vi "ExFilterWheelIN.vi"() -> ()   [LabVIEW 2010]
panel:
  out "Number of Filter Wheels":i16
  in  "?":bool
  out "Filter Wheel Open":bool
  out "Number Of Filters":i16=1 min=1 step=1
  in  "?":bool
  in  "?":bool
  out "Filter":i16=1 min=0 step=1
  in  "?":bool
  in  "?":bool
  in  "?":bool
  in  "Filter":i16=1 min=1 max=100 step=1
  out "error out":errorcluster
  in  "error in":errorcluster
  # "ExFilterWheelIN.vi (InSpectrum Only)\nThis example shows how access a filter wheel on the InSpectrum.\nNot all commands may be available for all filter wheels.\nNOTE: The properly configured spectrometer .ini file must be\npresent in the LabVIEW folder for spectrometer operation."
  # "Currently, there is only 1 filter wheel\navailable on the InSpectrum."
  # "The number of filters is set in the .ini file"
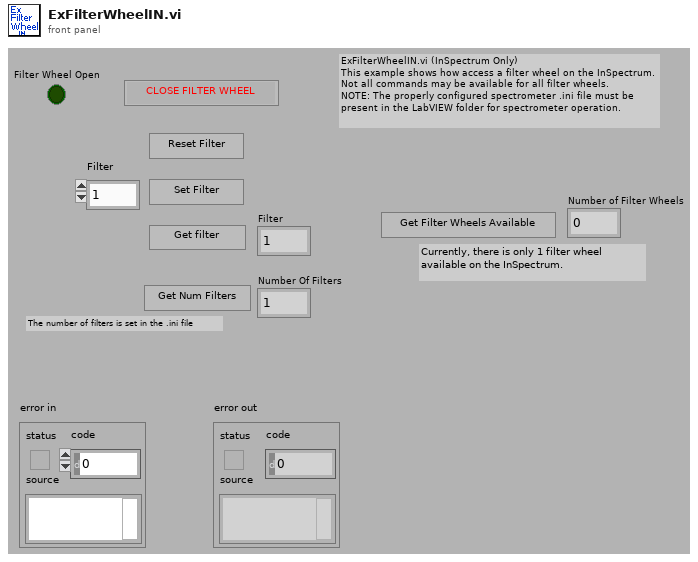
[diagram p1: front panel]
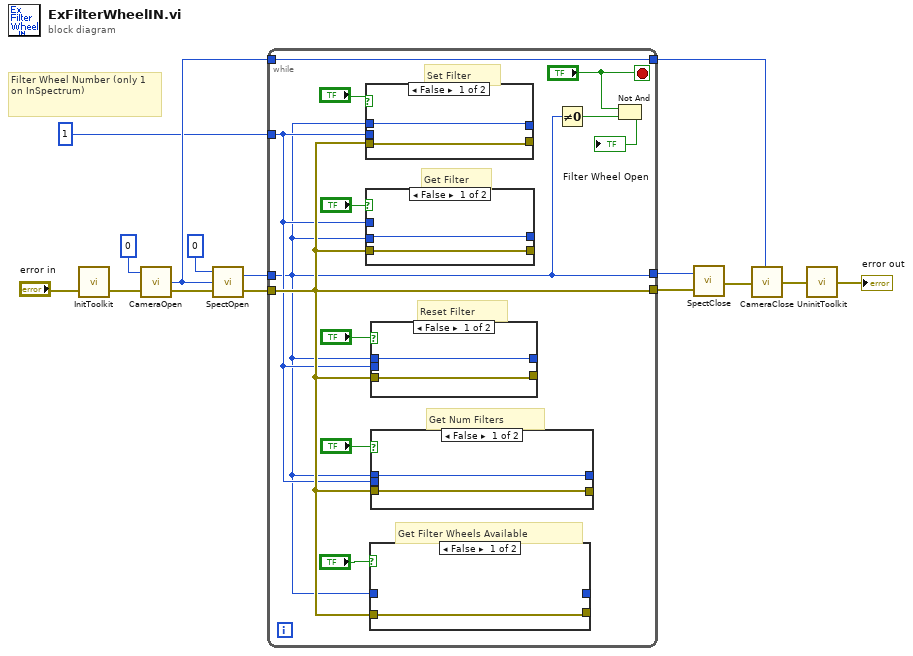
[diagram p0: block diagram]
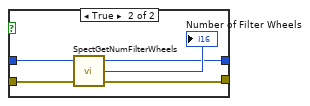
[diagram p2: hidden frame]
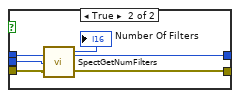
[diagram p3: hidden frame]
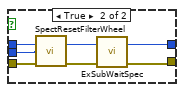
[diagram p4: hidden frame]
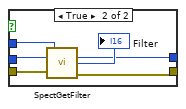
[diagram p5: hidden frame]
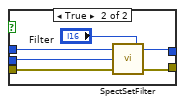
[diagram p6: hidden frame]
diagram:
  # "Filter Wheel Number (only 1 on InSpectrum)"
  n1 = call <userlib>:"InitToolkit.vi"("error in"="error in") -> ("error out"=w7:errorcluster)
  n2 = call <userlib>:"CameraOpen.vi"("error in"=w7, "Camera Device ID"=0) -> ("error out"=w6:errorcluster, "Camera Handle"=w2:u32)
  n3 = call <userlib>:"SpectOpen.vi"("error in"=w6, "Camera Handle"=w2, "Spectrometer ID"=0) -> ("error out"=w12:errorcluster, "Spectrometer Handle"=w9:u32)
  n4 = while {
    tunnel: w9 -> [w16]
    tunnel: w12 -> [w18]
    tunnel: [w16] -> w11
    tunnel: [w18] -> w10
    tunnel: w2 -> [w20]
    tunnel: [w20] -> w3
    tunnel: 1 -> [w17]
    stop <- "?" stop-if-true
    # "Get Filter Wheels Available"
    # "Get Num Filters"
    # "Get Filter"
    # "Set Filter"
    # "Reset Filter"
    n5 = case shown="False" "?" {
      tunnel: [w59 w66] -> _
      tunnel: [w60 w65] -> _
      tunnel: w16 -> [w60 w64]
      tunnel: w18 -> [w59 w63]
      tunnel: w17 -> [_ w62]
      frame False {
      }
      frame True {
        n6 = call <userlib>:"SpectSetFilter.vi"("Filter Number"="Filter", "error in"=w63, "Filter Wheel Number"=w62, "Spectrometer Handle"=w64) -> ("error out"=w66:errorcluster, "Spectrometer Handle"=w65:u32)
      }
    }
    n7 = case shown="False" "?" {
      tunnel: w16 -> [w52 w58]
      tunnel: w18 -> [w51 w57]
      tunnel: [w51 w56] -> _
      tunnel: [w52 w54] -> _
      tunnel: w17 -> [_ w53]
      frame False {
      }
      frame True {
        n8 = call <userlib>:"SpectGetFilter.vi"("error in"=w57, "Filter Wheel Number"=w53, "Spectrometer Handle"=w58) -> ("error out"=w56:errorcluster, "Filter Number"=→"Filter":i16, "Spectrometer Handle"=w54:u32)
      }
    }
    n9 = case shown="False" "?" {
      tunnel: w18 -> [w28 w32]
      tunnel: [w28 w33] -> _
      tunnel: w16 -> [_ w31]
      tunnel: [_ w29] -> _
      frame False {
      }
      frame True {
        n10 = call <userlib>:"SpectGetNumFilterWheels.vi"("error in"=w32, "Spectrometer Handle"=w31) -> ("error out"=w33:errorcluster, "Filter Number"=→"Number of Filter Wheels":i16, "Spectrometer Handle"=w29:u32)  [unwired: 1 in]
      }
    }
    n11 = case shown="False" "?" {
      tunnel: w18 -> [w42 w49]
      tunnel: w16 -> [w43 w50]
      tunnel: [w43 w47] -> _
      tunnel: [w42 w45] -> _
      tunnel: w17 -> [_ w44]
      frame False {
      }
      frame True {
        n12 = call <userlib>:"SpectResetFilterWheel.vi"("error in"=w49, "Filter Wheel"=w44, "Spectrometer Handle"=w50) -> ("error out"=w46:errorcluster, "Spectrometer Handle"=w48:u32)  [unwired: 1 in]
        n13 = call "ExSubWaitSpec.vi"("error in (no error)"=w46, "Spectrometer Handle"=w48) -> ("error out"=w45:errorcluster, "Spectrometer handle"=w47:u32)
      }
    }
    n14 = case shown="False" "?" {
      tunnel: w16 -> [w35 w40]
      tunnel: [w35 w39] -> _
      tunnel: w18 -> [w34 w38]
      tunnel: [w34 w37] -> _
      tunnel: w17 -> [_ w36]
      frame False {
      }
      frame True {
        n15 = call <userlib>:"SpectGetNumFilters.vi"("error in"=w38, "Filter Wheel"=w36, "Spectrometer Handle"=w40) -> ("error out"=w37:errorcluster, "Number of Filters"=→"Number Of Filters":i16, "Spectrometer Handle"=w39:u32)
      }
    }
    n16 = Not Equal To 0?(x=w16) -> (x != 0?=w23:bool)
    n17 = Not And(1:w23, 2:"?") -> (0:→"Filter Wheel Open":bool)
  }
  n18 = call <userlib>:"SpectClose.vi"("error in"=w10, "Spectrometer Handle"=w11) -> ("error out"=w5:errorcluster)
  n19 = call <userlib>:"CameraClose.vi"("error in"=w5, "Camera Handle"=w3) -> ("error out"=w4:errorcluster)
  n20 = call <userlib>:"UninitToolkit.vi"("error in"=w4) -> ("error out"=→"error out":errorcluster)
